vi "Log_Event.vi"(1 "Debug":bool, 2 "Event":cluster{string, string[], dbl[], dbl}) -> ()   [LabVIEW 2011]
doc: "This VI logs the execution of a given \"Event\". It will prepend a timestamp unless \"Debug\" is enabled, in which case it will prepend the given events total execution time."
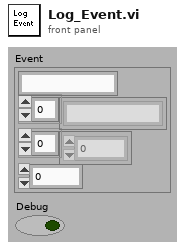
[diagram p1: front panel]
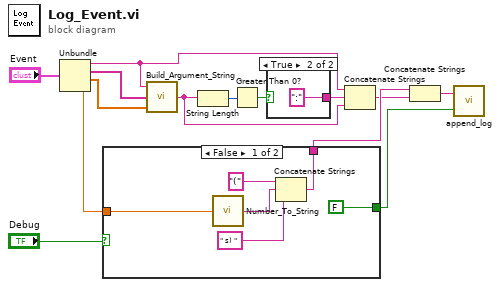
[diagram p0: block diagram]
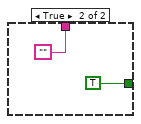
[diagram p2: hidden frame]
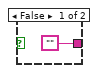
[diagram p3: hidden frame]
diagram:
  n1 = Unbundle("Event") -> (w14:string, w12:string[], w13:dbl[], w5:dbl)
  n2 = case shown="False" "Debug" {
    tunnel: [FALSE ("Prepend Timestamp (T)") TRUE ("Prepend Timestamp (T)")] -> w6
    tunnel: w5 -> [w17 _]
    tunnel: [w15 ""] -> w4
    frame False {
      n3 = call "Number_To_String.vi"("Number"=w17) -> ("String"=w18:string)
      n4 = Concatenate Strings("(", w18, " s) " ("string")) -> (w15:string)
    }
    frame True {
    }
  }
  n5 = call "Build_Argument_String.vi"("Flow Array"=w13, "Argument List"=w12, "Command"=w14) -> ("Argument String"=w10:string)
  n6 = String Length(string=w10) -> (length=w11:i32)
  n7 = Greater Than 0?(x=w11) -> (x > 0?=w9:bool)
  n8 = case shown="True" w9 {
    tunnel: ["" ":"] -> w8
    frame False {
    }
    frame True {
    }
  }
  n9 = Concatenate Strings(w14, w8, w10) -> (w3:string)
  n10 = Concatenate Strings(w4, w3) -> (w7:string)
  n11 = call "append_log.vi"("Prepend Timestamp (T)"=w6, "New Log String"=w7) -> ()  [unwired: 1 out]
